vi "naming.vi"() -> (6 "filename":string)   [LabVIEW 2012]
uses:
  variables/GlobalUI.vi
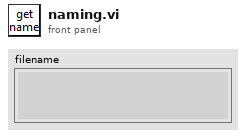
[diagram p1: front panel]
types:
  T1 = typedef "Filenaming.ctl" = enum16{"Image", "Just Description"}
  T2 = typedef "Scan Parameters.ctl" = cluster{"x pixels":i32, "x voltage min":dbl, "x voltage max":dbl, "y voltage min":dbl, "y voltage max":dbl, "fill frac":dbl, "Zoom":dbl, "BiDi":bool, "scan rate (ms/line)":dbl}
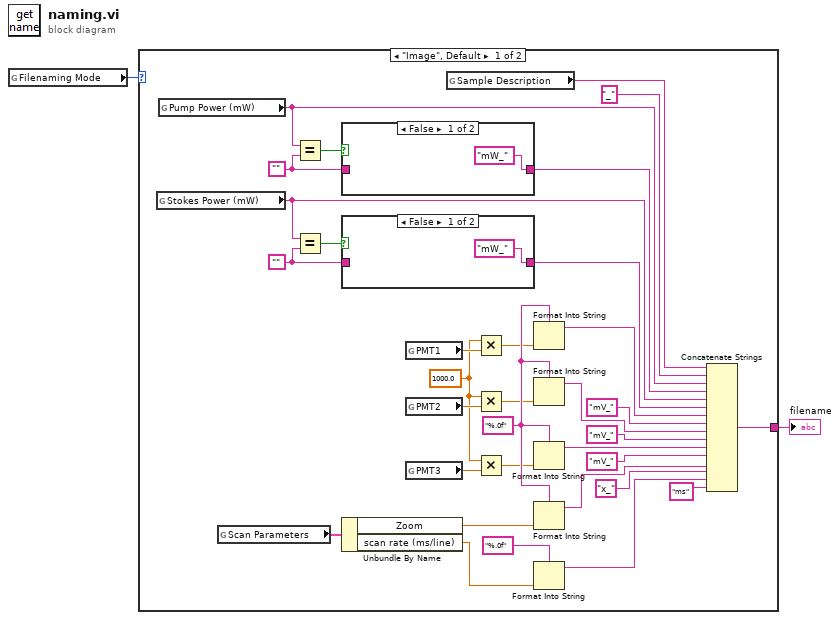
[diagram p0: block diagram]
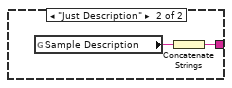
[diagram p4: hidden frame]
diagram:
  n1 = global read "GlobalUI.vi" "Filenaming Mode"() -> (w1:T1)
  n2 = case shown="\"Image\", Default" w1 {
    tunnel: [w4 w40] -> w2
    frame "Image", Default {
      w22 = ""
      w20 = ""
      w12 = 1000.0 ("x")
      w14 = "%.0f" ("format string")
      n3 = global read "GlobalUI.vi" "Stokes Power (mW)"() -> (w30:string)
      n4 = global read "GlobalUI.vi" "Pump Power (mW)"() -> (w31:string)
      n5 = global read "GlobalUI.vi" "Scan Parameters"() -> (w27:T2)
      n6 = Equal?(x=w31, y=w22) -> (x = y?=w23:bool)
      n7 = Equal?(x=w30, y=w20) -> (x = y?=w19:bool)
      n8 = case shown="False" w23 {
        tunnel: ["mW_" ("string") w37] -> w24
        tunnel: w22 -> [_ w37]
        frame False {
        }
        frame True {
        }
      }
      n9 = case shown="False" w19 {
        tunnel: ["mW_" ("string") w39] -> w21
        tunnel: w20 -> [_ w39]
        frame False {
        }
        frame True {
        }
      }
      n10 = Unbundle By Name(w27) -> ("Zoom"=w29:dbl, "scan rate (ms/line)"=w28:dbl)
      n11 = global read "GlobalUI.vi" "PMT1"() -> (w33:dbl)
      n12 = global read "GlobalUI.vi" "PMT2"() -> (w34:dbl)
      n13 = global read "GlobalUI.vi" "PMT3"() -> (w35:dbl)
      n14 = global read "GlobalUI.vi" "Sample Description"() -> (w32:string)
      n15 = Multiply(x=w12, y=w33) -> (x*y=w5:dbl)
      n16 = Multiply(x=w12, y=w34) -> (x*y=w6:dbl)
      n17 = Multiply(x=w12, y=w35) -> (x*y=w13:dbl)
      n18 = Format Into String(format string=w14, w5) -> (resulting string=w7:string)  [unwired: 2 in, 1 out]
      n19 = Format Into String(format string=w14, w6) -> (resulting string=w9:string)  [unwired: 2 in, 1 out]
      n20 = Format Into String(format string=w14, w13) -> (resulting string=w17:string)  [unwired: 2 in, 1 out]
      n21 = Format Into String(format string=w14, w29) -> (resulting string=w16:string)  [unwired: 2 in, 1 out]
      n22 = Format Into String(format string="%.0f", w28) -> (resulting string=w26:string)  [unwired: 2 in, 1 out]
      n23 = Concatenate Strings(w32, "_" ("string"), w31, w24, w30, w21, w7, "mV_" ("string"), w9, "mV_" ("string"), w17, "mV_" ("string"), w16, "x_" ("string"), w26, "ms" ("string")) -> (w4:string)
    }
    frame "Just Description" {
      n24 = global read "GlobalUI.vi" "Sample Description"() -> (w41:string)
      n25 = Concatenate Strings(w41) -> (w40:string)
    }
  }
  "filename" <- w2
